vi "http.put.vi"(6 "specific headers in":cluster{"header":string, "value":string}[](array[cluster]), 8 "error in":errorcluster, 9 "Body":string, 10 "Path":string, 11 "Nominal Client in":refnum<class "Nominal Client.lvclass">) -> (0 "error out":errorcluster, 2 "Response":string, 3 "Nominal Client out":refnum<class "Nominal Client.lvclass">)   [LabVIEW 2020, in "Nominal Client.lvclass"]
uses:
  Nominal Client.lvclass
  Nominal Client.lvclass/Nominal Client.ctl
  <vilib>/JDP Science/JSONtext/LVClass Serializer/JSONtext LVClass Serializer.lvclass
  submodules/reqwest-labview/lv-src/reqwest/reqwest.lvclass
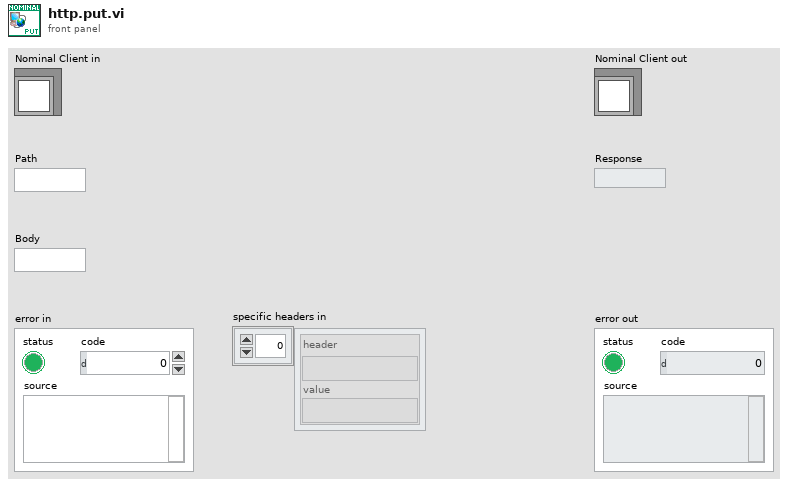
[diagram p1: front panel]
types:
  T1 = typedef "Nominal Client.lvclass/private_data.ctl" = cluster{"API Token":string, "workspace":refnum<class "workspace.lvclass">, "Available Workspaces":refnum<class "workspace.lvclass">[], "reqwest":refnum<class "reqwest.lvclass">, "timeout ms":i32}
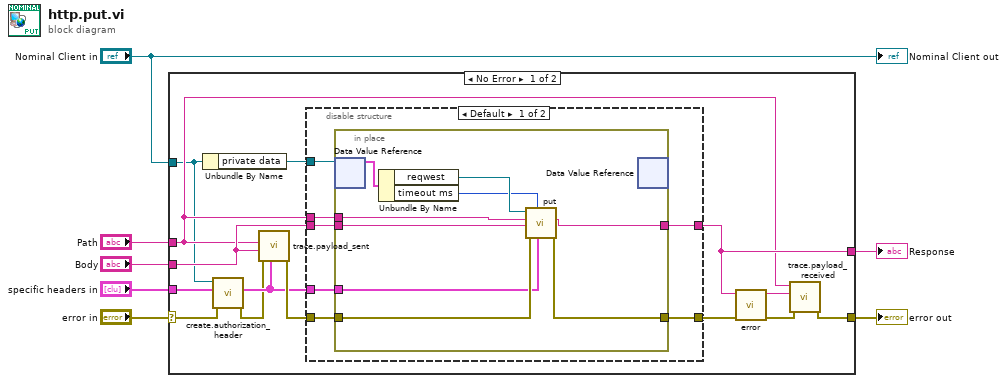
[diagram p0: block diagram]
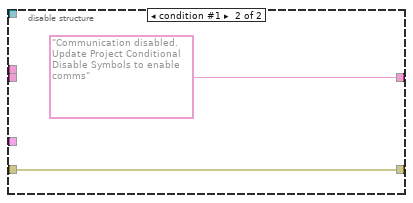
[diagram p2: hidden frame]
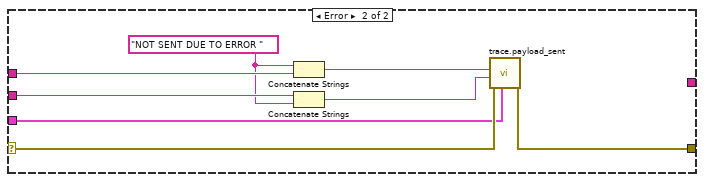
[diagram p3: hidden frame]
diagram:
  n1 = case shown="No Error" "error in" {
    selector: "error in" -> [w9 w42]
    tunnel: [w20 _] -> w7
    tunnel: "Body" -> [w18 w45]
    tunnel: "specific headers in" -> [w10 w40]
    tunnel: [w14 w41] -> w3
    tunnel: "Path" -> [w16 w46]
    tunnel: "Nominal Client in" -> [w12 _]
    frame No Error {
      n2 = Unbundle By Name(w12) -> ("private data"=w13:refnum<data-value>)
      n3 = call "create.authorization_header.vi"("error in"=w9, "specific headers in"=w10, "Nominal Client in"=w12) -> ("error out"=w8:errorcluster, "specific headers out"=w11:cluster{"header":string, "value":string}[])  [unwired: 6 in, 1 out]
      n4 = call "trace.payload_sent.vi"("Headers"=w11, "dataflow error in"=w8, "Request Body"=w18, "Path"=w16) -> ("dataflow error out"=w21:errorcluster)  [unwired: 7 in]
      n5 = disable-structure shown="Default" {
        disable-tunnel: [w28 "Communication disabled. Update Project Conditional Disable Symbols to enable comms" ("REST Response")] -> w20
        disable-tunnel: [w27 w39] -> w19
        disable-tunnel: w21 -> [w26 w39]
        disable-tunnel: w18 -> [w25 _]
        disable-tunnel: w11 -> [w24 _]
        disable-tunnel: w16 -> [w23 _]
        disable-tunnel: w13 -> [w22 _]
        frame condition #0 (active) {
          n6 = in-place {
            in-place-border: [w37] -> w28
            in-place-border: [w36] -> w27
            in-place-border: w26 -> [w35]
            in-place-border: w25 -> [w34]
            in-place-border: w24 -> [w31]
            in-place-border: w23 -> [w33]
            n7 = in-place-dvr #1(w22) -> (w32:T1)  [unwired: 1 out]
            n8 = Unbundle By Name(w32) -> ("reqwest"=w30:refnum<class "reqwest.lvclass">, "timeout ms"=w29:i32)
            n9 = call "put.vi"("request specific headers"=w31, "timeout (ms)"=w29, "error in (no error)"=w35, "request body"=w34, "path"=w33, "reqwest in"=w30) -> ("error out"=w36:errorcluster, "response"=w37:string)  [unwired: 3 in, 1 out]
            n10 = in-place-dvr #1() -> ()  [unwired: 1 in, 2 out]
          }
        }
        frame condition #1 {
        }
      }
      n11 = call "error.vi"("error in"=w19, "REST Response"=w20) -> ("error out"=w15:errorcluster, "Error Formatted Response"=w17:string)  [unwired: 8 in]
      n12 = call "trace.payload_received.vi"("dataflow error in"=w15, "Response"=w17, "Path"=w16) -> ("dataflow error out"=w14:errorcluster)  [unwired: 8 in]
    }
    frame Error {
      w44 = "NOT SENT DUE TO ERROR " ("string")
      n13 = Concatenate Strings(w44, w46) -> (w47:string)
      n14 = Concatenate Strings(w45, w44) -> (w43:string)
      n15 = call "trace.payload_sent.vi"("Headers"=w40, "dataflow error in"=w42, "Request Body"=w43, "Path"=w47) -> ("dataflow error out"=w41:errorcluster)  [unwired: 7 in]
    }
  }
  "error out" <- w3
  "Response" <- w7
  "Nominal Client out" <- "Nominal Client in"
